vi "CheckForEnabled.vi"(8 "error in (no error)":errorcluster, 11 "Mode":T1(ring)=enum."Auto Disabled") -> (0 "error out":errorcluster, 3 "Enabled":bool)   [LabVIEW 2012]
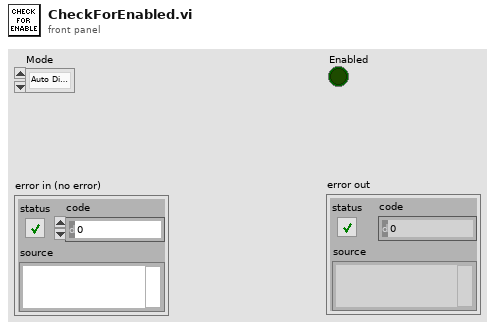
[diagram p1: front panel]
types:
  T1 = enum8{"Tele-Op Disabled", "Tele-Op Enabled", "Auto Disabled", "Auto Enabled", "Test Disabled", "Test Enabled", ""}
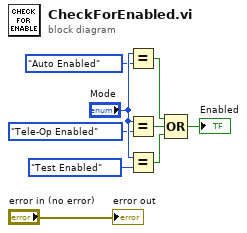
[diagram p0: block diagram]
diagram:
  n1 = Equal?(x="Mode", y=T1."Auto Enabled" ("Mode")) -> (x = y?=w6:bool)
  n2 = Equal?(x="Mode", y=T1."Tele-Op Enabled" ("Mode")) -> (x = y?=w8:bool)
  n3 = Equal?(x="Mode", y=T1."Test Enabled" ("Mode")) -> (x = y?=w7:bool)
  n4 = Compound Arithmetic op=OR(w6, w8, w7) -> (→"Enabled":bool)
  "error out" <- "error in (no error)"
